vi "Register Status Operations.vi"(8 "error in (no error)":errorcluster, 9 "SRE Bit(0)":i32, 10 "Register (0:*SRE)":i32(ring) items=["*SRE", "*CLS", "*OPC", "*WAI", "ESR2?", "*ESE?", "*ESR?", "*STB?"], 11 "VISA resource name":refnum<visa-resource-name>) -> (0 "error out":errorcluster, 2 "Register Status":i32, 3 "VISA resource name out":refnum<visa-resource-name>)   [LabVIEW 2020, in "Anritsu Signal Analyzer Series.lvlib"]
doc: "Sets or queries Registers."
uses:
  Anritsu Signal Analyzer Series.lvlib
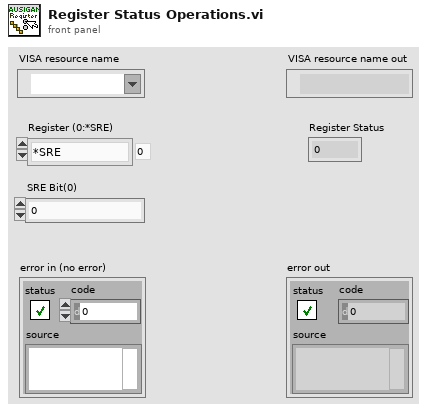
[diagram p1: front panel]
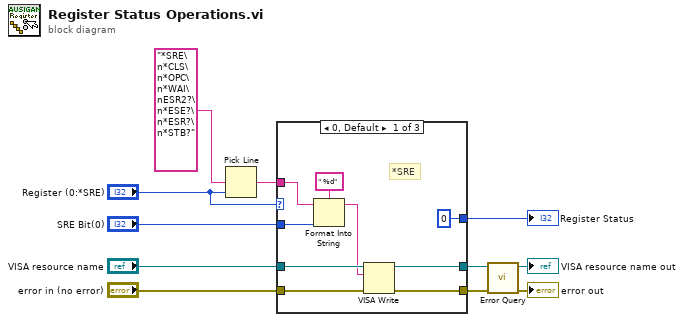
[diagram p0: block diagram]
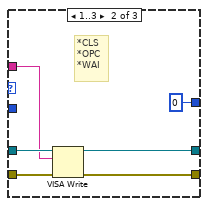
[diagram p2: hidden frame]
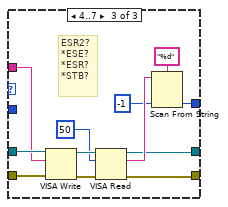
[diagram p3: hidden frame]
diagram:
  n1 = Pick Line(multi-line string="*SRE\n*CLS\n*OPC\n*WAI\nESR2?\n*ESE?\n*ESR?\n*STB?" ("_Command"), line index="Register (0:*SRE)") -> (output string=w5:string)  [unwired: 1 in]
  n2 = case shown="0, Default" "Register (0:*SRE)" {
    tunnel: "VISA resource name" -> [w20 w26 w33]
    tunnel: "error in (no error)" -> [w19 w25 w32]
    tunnel: w5 -> [w17 w24 w31]
    tunnel: [w16 w23 w30] -> w4
    tunnel: [w15 w22 w29] -> w3
    tunnel: "SRE Bit(0)" -> [w14 _ _]
    tunnel: [0 ("_Default") 0 ("_Default") w27] -> w1
    frame 0, Default {
      # "*SRE"
      n3 = Format Into String(format string=" %d" ("Format String"), initial string=w17, w14) -> (resulting string=w13:string)  [unwired: 1 in, 1 out]
      n4 = VISA Write(VISA resource name=w20, write buffer=w13, error in (no error)=w19) -> (VISA resource name out=w16:refnum<visa-resource-name>, error out=w15:errorcluster)  [unwired: 1 out]
    }
    frame 1..3 {
      # "*CLS\n*OPC\n*WAI"
      n5 = VISA Write(VISA resource name=w26, write buffer=w24, error in (no error)=w25) -> (VISA resource name out=w23:refnum<visa-resource-name>, error out=w22:errorcluster)  [unwired: 1 out]
    }
    frame 4..7 {
      # "ESR2?\n*ESE?\n*ESR?\n*STB?"
      n6 = VISA Write(VISA resource name=w33, write buffer=w31, error in (no error)=w32) -> (VISA resource name out=w38:refnum<visa-resource-name>, error out=w37:errorcluster)  [unwired: 1 out]
      n7 = VISA Read(VISA resource name=w38, byte count=u32 50 ("byte count (0)"), error in (no error)=w37) -> (VISA resource name out=w30:refnum<visa-resource-name>, read buffer=w35:string, error out=w29:errorcluster)  [unwired: 1 out]
      n8 = Scan From String(format string="%d" ("Format String"), input string=w35, default 1=-1 ("_Default")) -> (output 1=w27:i32)  [unwired: 2 in, 3 out]
    }
  }
  "Register Status" <- w1
  n9 = call "Error Query.vi"("error in (no error)"=w3, "VISA resource name"=w4) -> ("error out"=→"error out":errorcluster, "VISA resource name out"=→"VISA resource name out":refnum<visa-resource-name>)  [unwired: 6 in, 2 out]
